vi "Write Graph Data.vi"(10 "Graph Data":cluster{"Array":dbl[], "Array":dbl[]}[](array[cluster]), 11 "IMD in":refnum<class "IMD.lvclass">) -> (3 "IMD out":refnum<class "IMD.lvclass">)   [LabVIEW 2020, in "IMD.lvclass"]
uses:
  IMD.lvclass
  IMD.lvclass/IMD.ctl
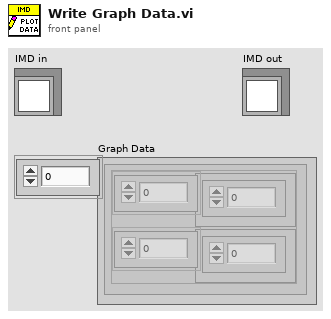
[diagram p1: front panel]
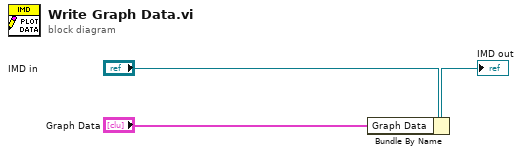
[diagram p0: block diagram]
diagram:
  n1 = Bundle By Name(cluster="IMD in", "Graph Data"="Graph Data") -> (→"IMD out":refnum<class "IMD.lvclass">)
